vi "Read Value.vi"(8 "Error In":errorcluster, 11 "Array In":refnum<class "Array.lvclass">) -> (0 "Error Out":errorcluster, 2 "Value":refnum<class "Abstract.lvclass">[](array[class]), 3 "Array Out":refnum<class "Array.lvclass">)   [LabVIEW 2018, in "Toolkit.lvlib" / "Data.lvlib" / "Array.lvclass"]
uses:
  Array.lvclass
  Abstract/Abstract.lvclass
  Array.lvclass/Array.ctl
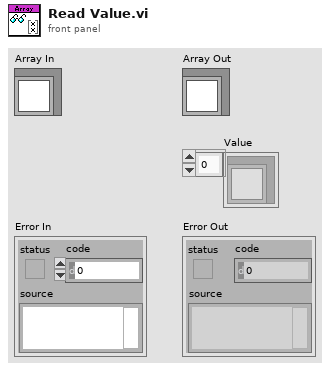
[diagram p1: front panel]
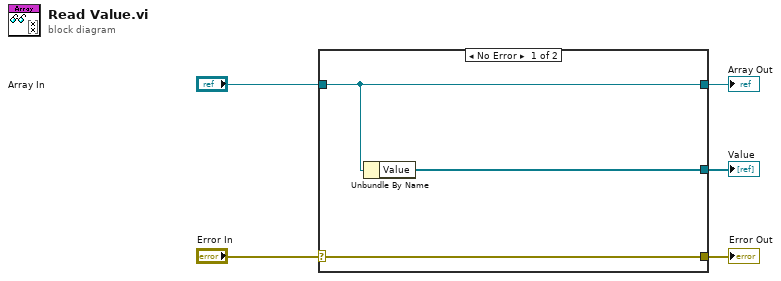
[diagram p0: block diagram]
diagram:
  n1 = case shown="No Error" "Error In" {
    selector: "Error In" -> [w8 w9]
    tunnel: [w8 w9] -> w4
    tunnel: [w7 w10] -> w2
    tunnel: "Array In" -> [w7 w10]
    tunnel: [w6 _] -> w1
    frame No Error {
      n2 = Unbundle By Name(w7) -> ("Value"=w6:refnum<class "Abstract.lvclass">[])
    }
    frame Error {
    }
  }
  "Error Out" <- w4
  "Array Out" <- w2
  "Value" <- w1
